vi "Parse.vi"(8 "Error In":errorcluster, 11 "object in":refnum<class "2024_11.lvclass">) -> (0 "Error Out":errorcluster, 3 "object out":refnum<class "2024_11.lvclass">)   [LabVIEW 2023, in "2024_11.lvclass"]
uses:
  2024_11.lvclass
  2024_11.lvclass/2024_11.ctl
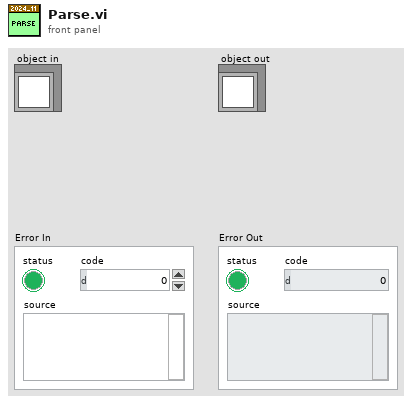
[diagram p1: front panel]
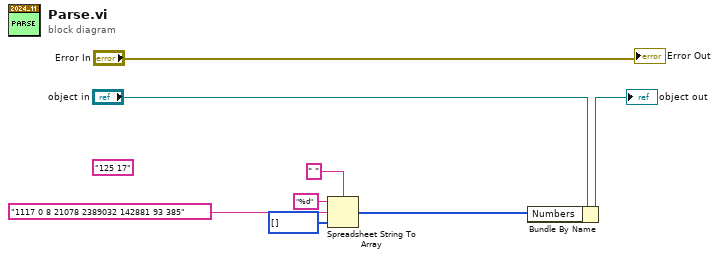
[diagram p0: block diagram]
diagram:
  (unwired) "125 17" ("PuzzleInput")
  n1 = Spreadsheet String To Array(delimiter (Tab)=" ", format string="%d", spreadsheet string="1117 0 8 21078 2389032 142881 93 385" ("PuzzleInput"), array type (2D Dbl)=u64[] []) -> (array=w2:u64[])
  n2 = Bundle By Name(cluster="object in", "Numbers"=w2) -> (→"object out":refnum<class "2024_11.lvclass">)
  "Error Out" <- "Error In"
